vi "camera-make_read-frame.vi"(11 "Address":string) -> (3 "Serial String":string)   [LabVIEW 2012]
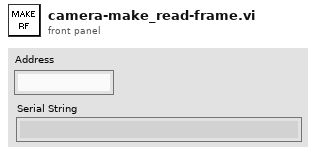
[diagram p1: front panel]
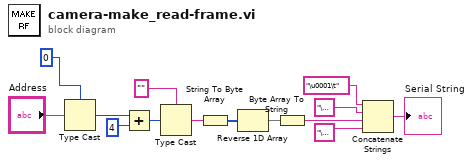
[diagram p0: block diagram]
diagram:
  n1 = Type Cast(type=u32 0 ("y"), x="Address") -> (*(type *) &x=w11:u32)
  n2 = Add(x=w11, y=u32 4) -> (x+y=w10:u32)
  n3 = Type Cast(type="", x=w10) -> (*(type *) &x=w6:string)
  n4 = String To Byte Array(string=w6) -> (unsigned byte array=w8:u8[])
  n5 = Reverse 1D Array(array=w8) -> (reversed array=w7:u8[])
  n6 = Byte Array To String(unsigned byte array=w7) -> (string=w5:string)
  n7 = Concatenate Strings("\u0001\t", "\u0004" ("string"), w5, "\u0003") -> (→"Serial String":string)
